vi "interpretatie positie t.o.v lijn (SubVI).vi"(0 "Array in":i32[](array[numeric])) -> (2 "Boolean 8":bool, 3 "Boolean 9":bool, 4 "Boolean":bool, 6 "Boolean 5":bool, 8 "Boolean 7":bool, 10 "Boolean 3":bool, 12 "Boolean 6":bool, 13 "Boolean 4":bool, 14 "Boolean 2":bool)   [LabVIEW 2019]
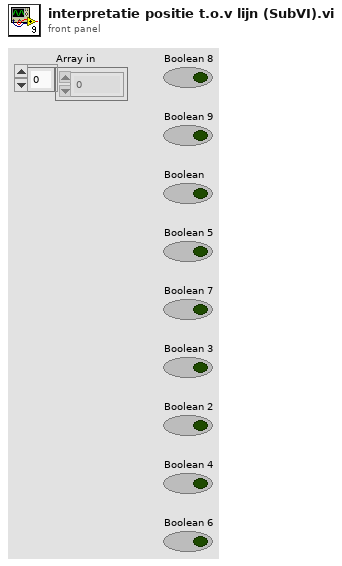
[diagram p1: front panel]
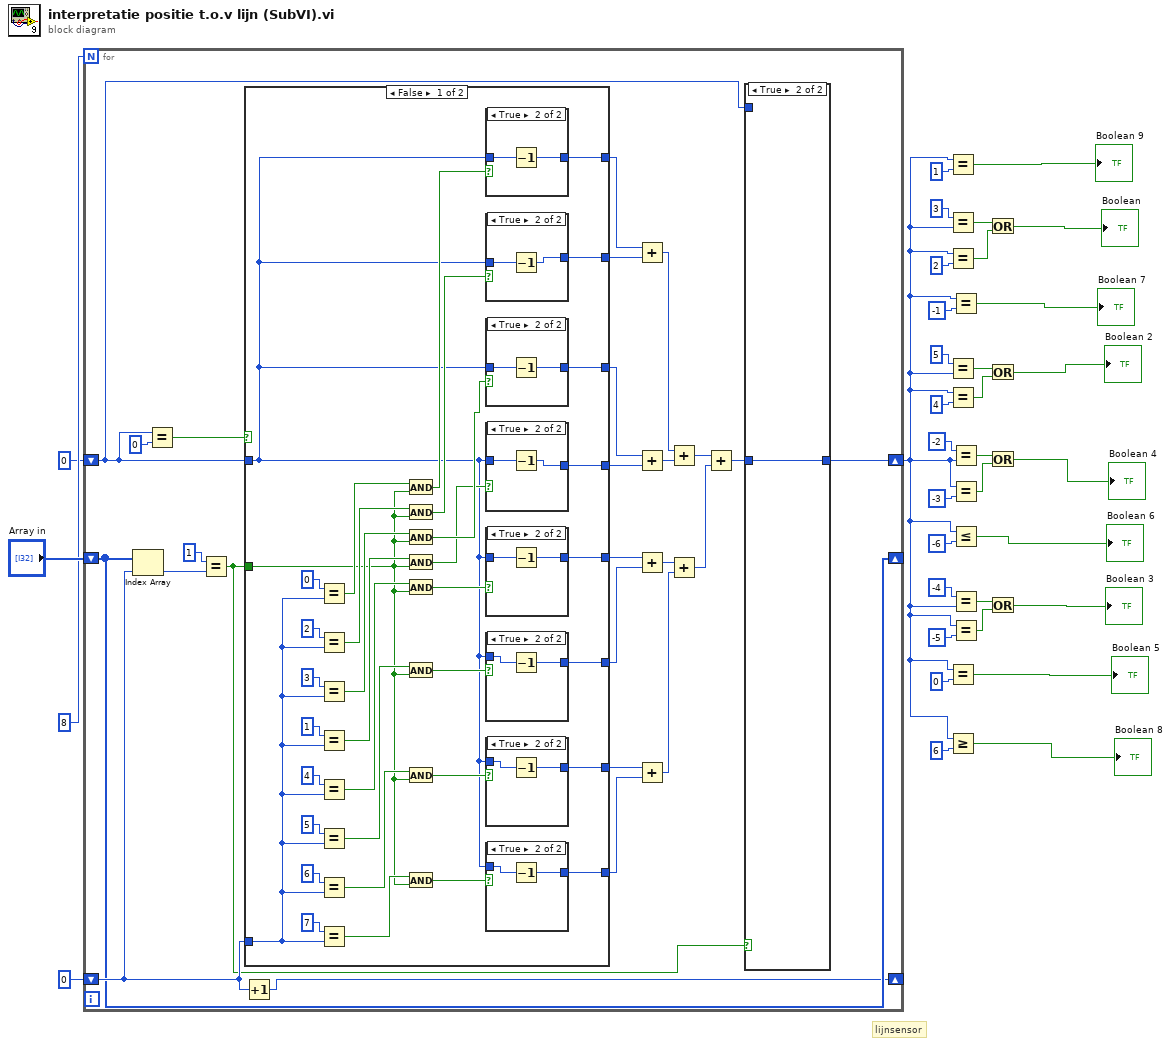
[diagram p0: block diagram]
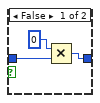
[diagram p3: hidden frame]
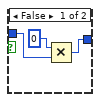
[diagram p4: hidden frame]
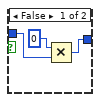
[diagram p5: hidden frame]
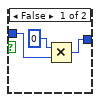
[diagram p6: hidden frame]
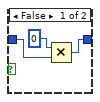
[diagram p7: hidden frame]
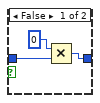
[diagram p8: hidden frame]
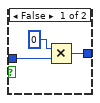
[diagram p9: hidden frame]
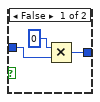
[diagram p10: hidden frame]
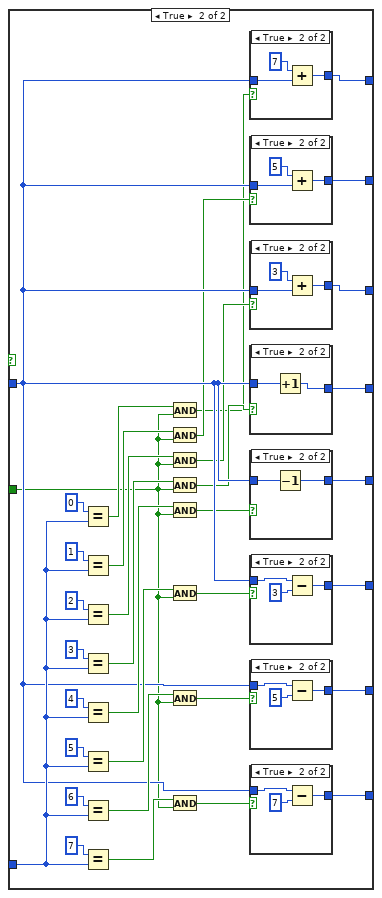
[diagram p11: hidden frame]
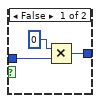
[diagram p12: hidden frame]
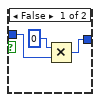
[diagram p13: hidden frame]
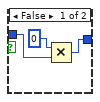
[diagram p14: hidden frame]
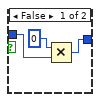
[diagram p15: hidden frame]
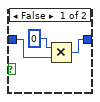
[diagram p16: hidden frame]
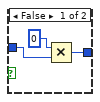
[diagram p17: hidden frame]
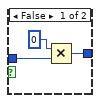
[diagram p18: hidden frame]
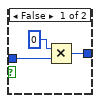
[diagram p19: hidden frame]
diagram:
  # "lijnsensor"
  n1 = for {
    N: 8 -> [_]
    shift-right: [w46] -> _
    shift-left: 0 -> [w60]
    shift-right: [w38] -> w31
    shift-left: 0 -> [w39]
    shift-right: [w51] -> _
    shift-left: "Array in" -> [w51]
    n2 = Index Array(array=w51, index=w60) -> (element=w50:i32)
    n3 = Equal?(x=w39, y=0) -> (x = y?=w47:bool)
    n4 = Equal?(x=1, y=w50) -> (x = y?=w37:bool)
    n5 = Increment(x=w60) -> (x+1=w46:i32)
    n6 = case shown="False" w47 {
      tunnel: w60 -> [w70 w156]
      tunnel: [w64 w155] -> w59
      tunnel: [w71 w154] -> w58
      tunnel: [w72 w153] -> w57
      tunnel: [w73 w152] -> w56
      tunnel: w39 -> [w63 w151]
      tunnel: w37 -> [w69 w142]
      tunnel: [w67 w141] -> w45
      tunnel: [w68 w140] -> w44
      tunnel: [w65 w139] -> w42
      tunnel: [w66 w138] -> w41
      frame False {
        n7 = Equal?(x=0, y=w70) -> (x = y?=w90:bool)
        n8 = Equal?(x=2, y=w70) -> (x = y?=w96:bool)
        n9 = Equal?(x=3, y=w70) -> (x = y?=w97:bool)
        n10 = Equal?(x=1, y=w70) -> (x = y?=w82:bool)
        n11 = Equal?(x=4, y=w70) -> (x = y?=w94:bool)
        n12 = Equal?(x=5, y=w70) -> (x = y?=w95:bool)
        n13 = Equal?(x=6, y=w70) -> (x = y?=w93:bool)
        n14 = Equal?(x=7, y=w70) -> (x = y?=w92:bool)
        n15 = And(x=w90, y=w69) -> (x .and. y?=w74:bool)
        n16 = And(x=w96, y=w69) -> (x .and. y?=w76:bool)
        n17 = And(x=w97, y=w69) -> (x .and. y?=w77:bool)
        n18 = And(x=w82, y=w69) -> (x .and. y?=w75:bool)
        n19 = And(x=w94, y=w69) -> (x .and. y?=w78:bool)
        n20 = And(x=w95, y=w69) -> (x .and. y?=w79:bool)
        n21 = And(x=w93, y=w69) -> (x .and. y?=w80:bool)
        n22 = And(x=w92, y=w69) -> (x .and. y?=w81:bool)
        n23 = case shown="True" w74 {
          tunnel: [w99 w102] -> w68
          tunnel: w63 -> [w98 w101]
          frame False {
            n24 = Multiply(x=0, y=w98) -> (x*y=w99:i32)
          }
          frame True {
            n25 = Decrement(x=w101) -> (x-1=w102:i32)
          }
        }
        n26 = case shown="True" w76 {
          tunnel: [w130 w131] -> w67
          tunnel: w63 -> [w129 w132]
          frame False {
            n27 = Multiply(x=0, y=w129) -> (x*y=w130:i32)
          }
          frame True {
            n28 = Decrement(x=w132) -> (x-1=w131:i32)
          }
        }
        n29 = case shown="True" w77 {
          tunnel: [w124 w127] -> w66
          tunnel: w63 -> [w123 w126]
          frame False {
            n30 = Multiply(x=0, y=w123) -> (x*y=w124:i32)
          }
          frame True {
            n31 = Decrement(x=w126) -> (x-1=w127:i32)
          }
        }
        n32 = case shown="True" w75 {
          tunnel: [w134 w137] -> w65
          tunnel: w63 -> [w133 w136]
          frame False {
            n33 = Multiply(x=0, y=w133) -> (x*y=w134:i32)
          }
          frame True {
            n34 = Decrement(x=w136) -> (x-1=w137:i32)
          }
        }
        n35 = case shown="True" w78 {
          tunnel: [w119 w122] -> w64
          tunnel: w63 -> [w118 w121]
          frame False {
            n36 = Multiply(x=0, y=w118) -> (x*y=w119:i32)
          }
          frame True {
            n37 = Decrement(x=w121) -> (x-1=w122:i32)
          }
        }
        n38 = case shown="True" w79 {
          tunnel: [w109 w112] -> w71
          tunnel: w63 -> [w108 w111]
          frame False {
            n39 = Multiply(x=0, y=w108) -> (x*y=w109:i32)
          }
          frame True {
            n40 = Decrement(x=w111) -> (x-1=w112:i32)
          }
        }
        n41 = case shown="True" w80 {
          tunnel: [w114 w117] -> w72
          tunnel: w63 -> [w113 w116]
          frame False {
            n42 = Multiply(x=0, y=w113) -> (x*y=w114:i32)
          }
          frame True {
            n43 = Decrement(x=w116) -> (x-1=w117:i32)
          }
        }
        n44 = case shown="True" w81 {
          tunnel: [w103 w107] -> w73
          tunnel: w63 -> [w104 w106]
          frame False {
            n45 = Multiply(x=0, y=w104) -> (x*y=w103:i32)
          }
          frame True {
            n46 = Decrement(x=w106) -> (x-1=w107:i32)
          }
        }
      }
      frame True {
        n47 = Equal?(x=0, y=w156) -> (x = y?=w165:bool)
        n48 = Equal?(x=1, y=w156) -> (x = y?=w157:bool)
        n49 = Equal?(x=2, y=w156) -> (x = y?=w171:bool)
        n50 = Equal?(x=3, y=w156) -> (x = y?=w172:bool)
        n51 = Equal?(x=4, y=w156) -> (x = y?=w169:bool)
        n52 = Equal?(x=5, y=w156) -> (x = y?=w170:bool)
        n53 = Equal?(x=6, y=w156) -> (x = y?=w168:bool)
        n54 = Equal?(x=7, y=w156) -> (x = y?=w167:bool)
        n55 = And(x=w165, y=w142) -> (x .and. y?=w143:bool)
        n56 = And(x=w157, y=w142) -> (x .and. y?=w144:bool)
        n57 = And(x=w171, y=w142) -> (x .and. y?=w145:bool)
        n58 = And(x=w172, y=w142) -> (x .and. y?=w146:bool)
        n59 = And(x=w169, y=w142) -> (x .and. y?=w147:bool)
        n60 = And(x=w170, y=w142) -> (x .and. y?=w148:bool)
        n61 = And(x=w168, y=w142) -> (x .and. y?=w149:bool)
        n62 = And(x=w167, y=w142) -> (x .and. y?=w150:bool)
        n63 = case shown="True" w143 {
          tunnel: w151 -> [w173 w177]
          tunnel: [w174 w176] -> w140
          frame False {
            n64 = Multiply(x=0, y=w173) -> (x*y=w174:i32)
          }
          frame True {
            n65 = Add(x=7, y=w177) -> (x+y=w176:i32)
          }
        }
        n66 = case shown="True" w144 {
          tunnel: w151 -> [w213 w216]
          tunnel: [w214 w217] -> w141
          frame False {
            n67 = Multiply(x=0, y=w213) -> (x*y=w214:i32)
          }
          frame True {
            n68 = Add(x=5, y=w216) -> (x+y=w217:i32)
          }
        }
        n69 = case shown="True" w145 {
          tunnel: w151 -> [w207 w211]
          tunnel: [w208 w210] -> w138
          frame False {
            n70 = Multiply(x=0, y=w207) -> (x*y=w208:i32)
          }
          frame True {
            n71 = Add(x=3, y=w211) -> (x+y=w210:i32)
          }
        }
        n72 = case shown="True" w146 {
          tunnel: w151 -> [w203 w206]
          tunnel: [w202 w205] -> w139
          frame False {
            n73 = Multiply(x=0, y=w203) -> (x*y=w202:i32)
          }
          frame True {
            n74 = Increment(x=w206) -> (x+1=w205:i32)
          }
        }
        n75 = case shown="True" w147 {
          tunnel: w151 -> [w197 w201]
          tunnel: [w198 w200] -> w155
          frame False {
            n76 = Multiply(x=0, y=w197) -> (x*y=w198:i32)
          }
          frame True {
            n77 = Decrement(x=w201) -> (x-1=w200:i32)
          }
        }
        n78 = case shown="True" w148 {
          tunnel: w151 -> [w186 w188]
          tunnel: [w185 w190] -> w154
          frame False {
            n79 = Multiply(x=0, y=w186) -> (x*y=w185:i32)
          }
          frame True {
            n80 = Subtract(x=w188, y=3) -> (x-y=w190:i32)
          }
        }
        n81 = case shown="True" w149 {
          tunnel: w151 -> [w192 w194]
          tunnel: [w191 w195] -> w153
          frame False {
            n82 = Multiply(x=0, y=w192) -> (x*y=w191:i32)
          }
          frame True {
            n83 = Subtract(x=w194, y=5) -> (x-y=w195:i32)
          }
        }
        n84 = case shown="True" w150 {
          tunnel: w151 -> [w179 w182]
          tunnel: [w180 w183] -> w152
          frame False {
            n85 = Multiply(x=0, y=w179) -> (x*y=w180:i32)
          }
          frame True {
            n86 = Subtract(x=w182, y=7) -> (x-y=w183:i32)
          }
        }
      }
    }
    n87 = Add(x=w44, y=w45) -> (x+y=w43:i32)
    n88 = Add(x=w41, y=w42) -> (x+y=w40:i32)
    n89 = Add(x=w59, y=w58) -> (x+y=w54:i32)
    n90 = Add(x=w57, y=w56) -> (x+y=w55:i32)
    n91 = Add(x=w43, y=w40) -> (x+y=w53:i32)
    n92 = Add(x=w54, y=w55) -> (x+y=w52:i32)
    n93 = Add(x=w53, y=w52) -> (x+y=w36:i32)
    n94 = case shown="True" w37 {
      tunnel: w39 -> [w61 _]
      tunnel: [w61 w62] -> w38
      tunnel: w36 -> [_ w62]
      frame False {
      }
      frame True {
      }
    }
  }
  n95 = Equal?(x=w31, y=1) -> (x = y?=→"Boolean 9":bool)
  n96 = Equal?(x=3, y=w31) -> (x = y?=w14:bool)
  n97 = Equal?(x=w31, y=2) -> (x = y?=w13:bool)
  n98 = Equal?(x=5, y=w31) -> (x = y?=w10:bool)
  n99 = Equal?(x=w31, y=4) -> (x = y?=w9:bool)
  n100 = Equal?(x=w31, y=0) -> (x = y?=→"Boolean 5":bool)
  n101 = Greater Or Equal?(x=w31, y=6) -> (x >= y?=→"Boolean 8":bool)
  n102 = Equal?(x=w31, y=-1) -> (x = y?=→"Boolean 7":bool)
  n103 = Equal?(x=-2, y=w31) -> (x = y?=w19:bool)
  n104 = Equal?(x=w31, y=-3) -> (x = y?=w18:bool)
  n105 = Less Or Equal?(x=w31, y=-6) -> (x <= y?=→"Boolean 6":bool)
  n106 = Equal?(x=-4, y=w31) -> (x = y?=w23:bool)
  n107 = Equal?(x=w31, y=-5) -> (x = y?=w22:bool)
  n108 = Or(x=w14, y=w13) -> (x .or. y?=→"Boolean":bool)
  n109 = Or(x=w10, y=w9) -> (x .or. y?=→"Boolean 2":bool)
  n110 = Or(x=w19, y=w18) -> (x .or. y?=→"Boolean 4":bool)
  n111 = Or(x=w23, y=w22) -> (x .or. y?=→"Boolean 3":bool)
